vi "Waveform Chart, Zoom in on Pulse.vi"(8 "error in":errorcluster, 9 "XScale:Max":dbl=0.3 format="%.3p", 10 "XScale:Min":dbl=0.2 format="%.3p", 11 "WFGraph ref":refnum<vi>) -> (0 "error out":errorcluster, 3 "WFGraph ref dup":refnum<vi>)   [LabVIEW 2010]
doc: "This function zooms in on a pulse by changing the x-axis scale factor, then setting the y-scale factor to auto."
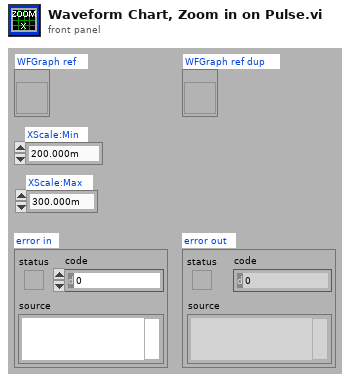
[diagram p1: front panel]
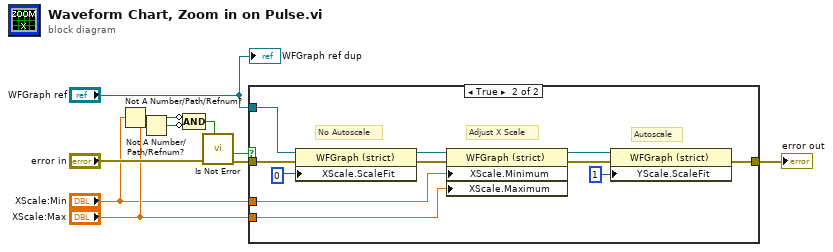
[diagram p0: block diagram]
diagram:
  n1 = Not A Number/Path/Refnum?(number/path/refnum="XScale:Min") -> (NaN/Path/Refnum?=w5:bool)
  n2 = Not A Number/Path/Refnum?(number/path/refnum="XScale:Max") -> (NaN/Path/Refnum?=w1:bool)
  n3 = Compound Arithmetic op=AND(invert w5, invert w1) -> (w2:bool)
  n4 = call "Is Not Error.vi"("enable (T)"=w2, "error in"="error in") -> ("error out"=w6:errorcluster, "ready"=w7:bool)  [unwired: 4 in, 1 out]
  n5 = case shown="True" w7 {
    tunnel: [w11 w16] -> w10
    tunnel: "WFGraph ref" -> [_ w22]
    tunnel: "XScale:Min" -> [_ w19]
    tunnel: "XScale:Max" -> [_ w18]
    tunnel: w6 -> [w11 w12]
    frame False {
    }
    frame True {
      # "Autoscale"
      # "Adjust X Scale"
      # "No Autoscale"
      n6 = property class="WFGraph (strict)"(reference=w22, error in=w12, "XScale.ScaleFit"=u8 0 ("Y Scale.Scale Fit")) -> (reference out=w20:refnum<vi>, error out=w21:errorcluster)
      n7 = property class="WFGraph (strict)"(reference=w20, error in=w21, "XScale.Minimum"=w19, "XScale.Maximum"=w18) -> (reference out=w13:refnum<vi>, error out=w14:errorcluster)
      n8 = property class="WFGraph (strict)"(reference=w13, error in=w14, "YScale.ScaleFit"=u8 1 ("Y Scale.Scale Fit")) -> (error out=w16:errorcluster)  [unwired: 1 out]
    }
  }
  "error out" <- w10
  "WFGraph ref dup" <- "WFGraph ref"
